vi "Kernel.vi"(0 "ref in":refnum<class "G#StaticClass.lvclass">, 1 "object name":string, 2 "option 1":bool, 3 "option 2":bool, 4 "depth":i32, 5 "error in (no error)":errorcluster, 6 "state":T3, 7 "option 3":bool, 8 "attributes in":variant[](array[variant]), 10 "class attributes in":variant[](array[variant])) -> (11 "class attributes out":variant[](array[variant]), 12 "class hierarchy":T1[](array[typedef]), 13 "attributes out":variant[](array[variant]), 14 "ref out":refnum<class "G#StaticClass.lvclass">, 15 "AttributeRefs":u32[](array[numeric]), 16 "static attribute ref":u32, 17 "output 1":bool, 18 "output 2":bool, 19 "error out":errorcluster)   [LabVIEW 2017, in "G#StaticClass.lvclass"]
doc: "Class kernel, creates and destroys the data value references of the class."
uses:
  G#StaticClass.lvclass
  <vilib>/addons/_AddQ/G#Object/utils/G#Object_State.ctl
  C:/Program Files/National Instruments/LabVIEW 2017/vi.lib/addons/_AddQ/G#Object/G#Object.lvclass
  <vilib>/addons/_AddQ/G#Object/utils/G#Object_ClassHierarchy.ctl
  protected/ClassAttributes.ctl
  ClassAttributesRef.ctl
  <vilib>/addons/_AddQ/G#Object/G#Object.lvclass
panel:
  in  "class attributes type":T2
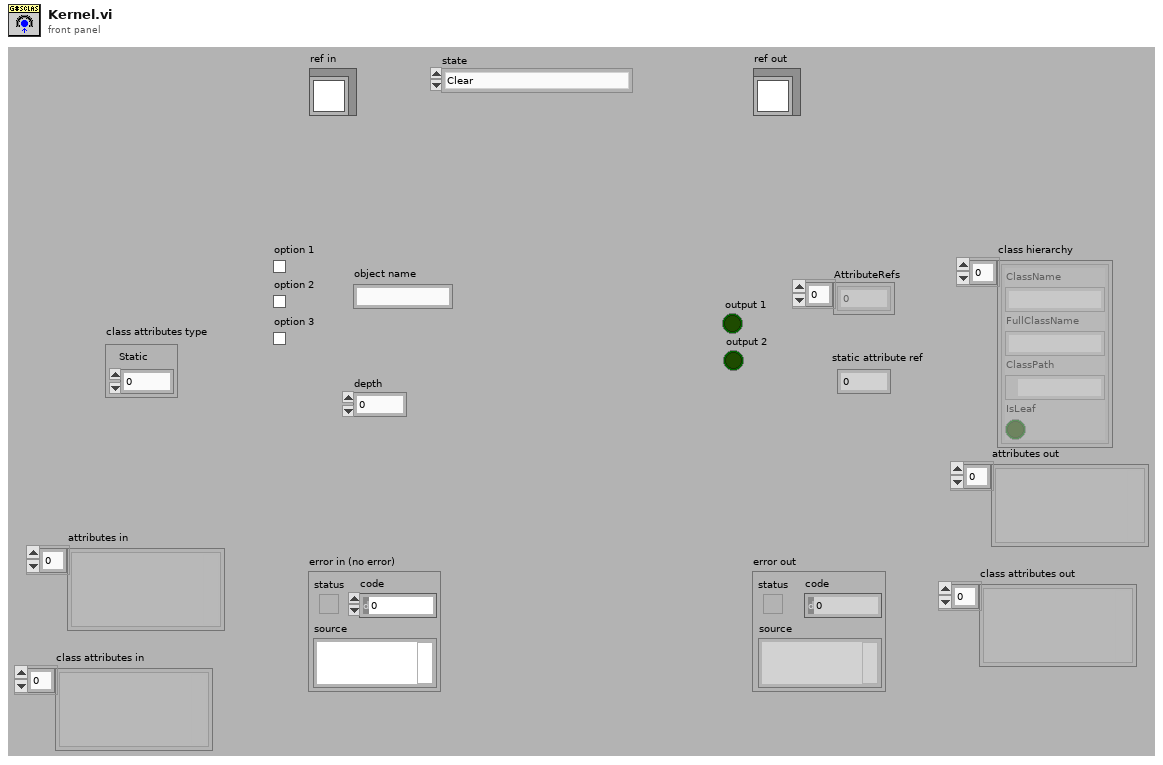
[diagram p1: front panel]
types:
  T1 = typedef "G#Object.lvclass/G#Object_ClassHierarchy.ctl" = cluster{"ClassName":string, "FullClassName":string, "ClassPath":path, "IsLeaf":bool}
  T2 = typedef "G#StaticClass.lvclass/ClassAttributes.ctl" = cluster{"Static":i32}
  T3 = typedef "G#Object.lvclass/G#Object_State.ctl" = enum16{"Clear", "Create", "Delete", "Get class attributes", "Class hierarchy", "Get attribute value", "Set attribute value"}
  T4 = typedef "G#StaticClass.lvclass/ClassAttributesRef.ctl" = refnum<data-value>
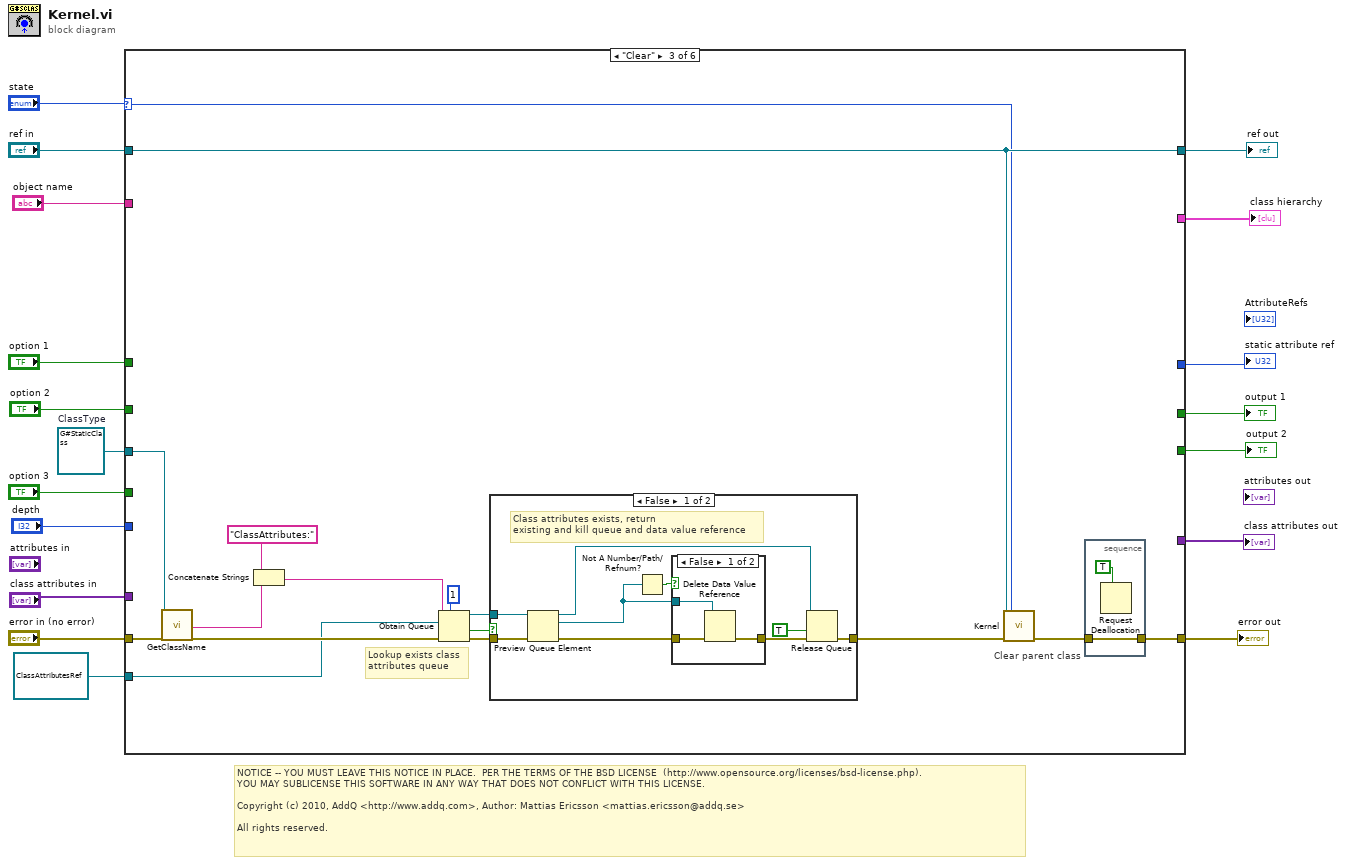
[diagram p0: block diagram]
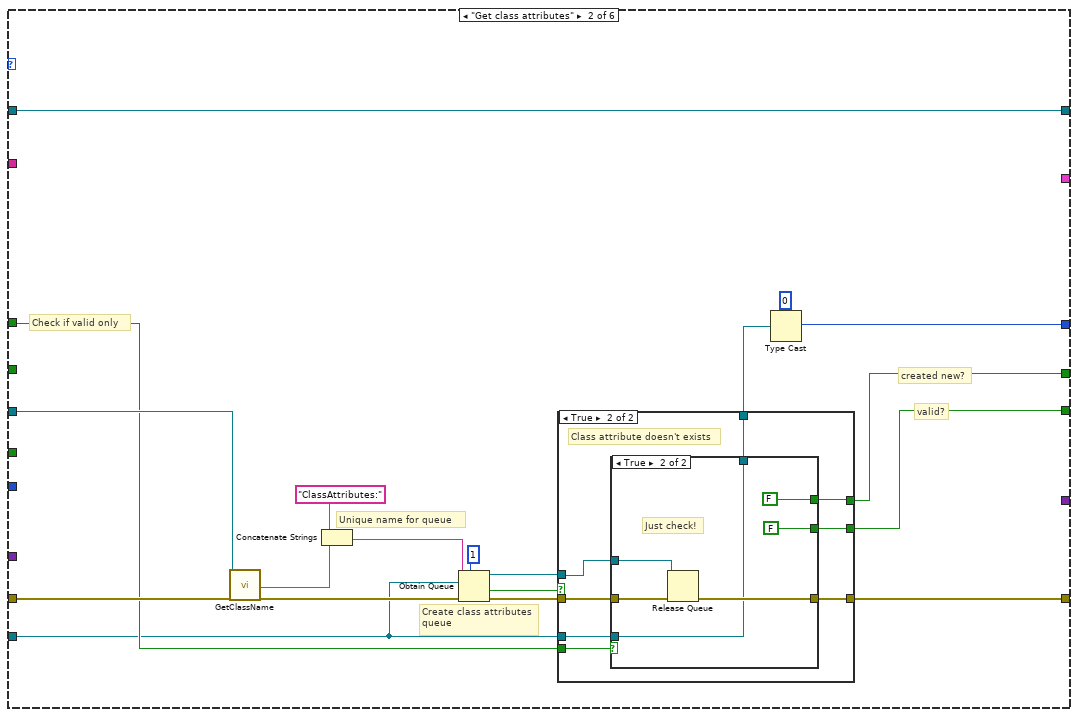
[diagram p3: hidden frame]
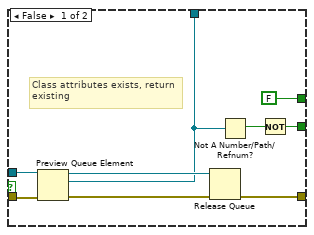
[diagram p4: hidden frame]
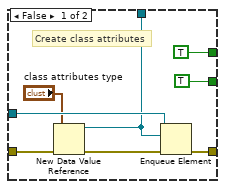
[diagram p5: hidden frame]
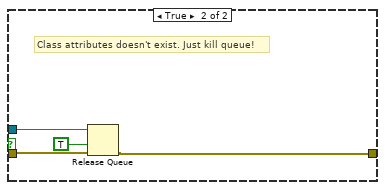
[diagram p7: hidden frame]
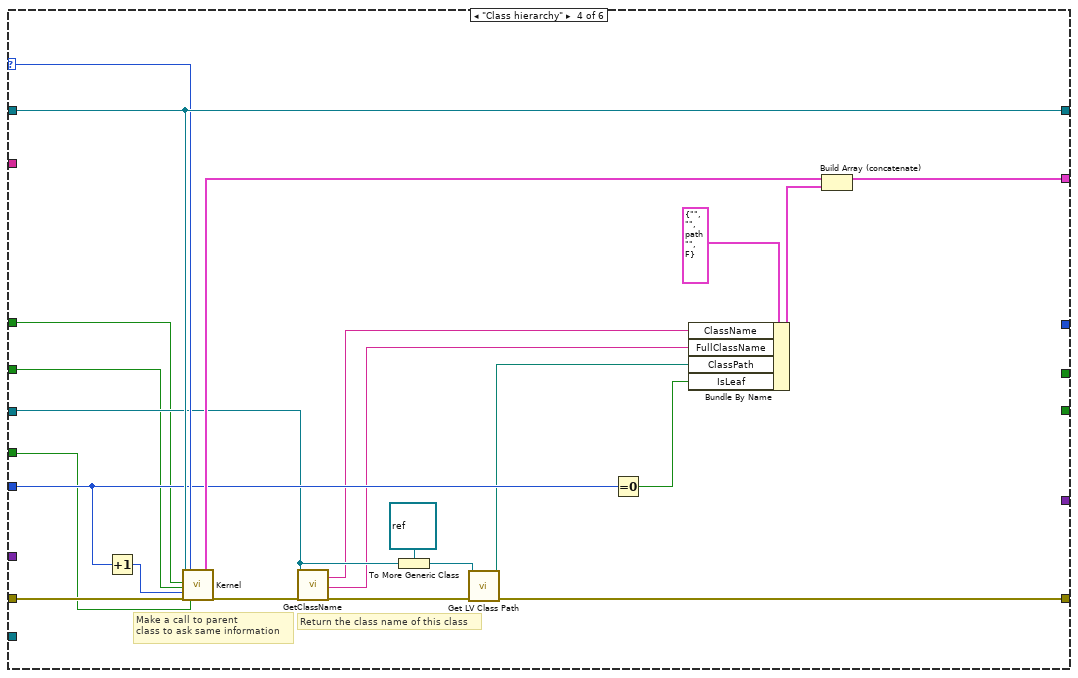
[diagram p8: hidden frame]
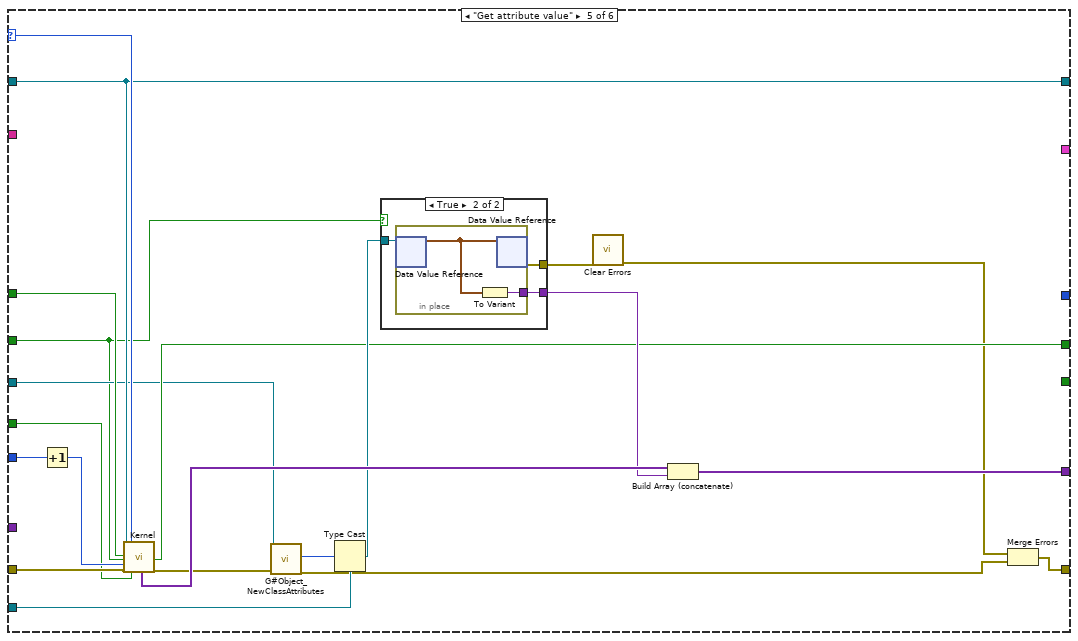
[diagram p9: hidden frame]
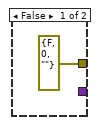
[diagram p10: hidden frame]
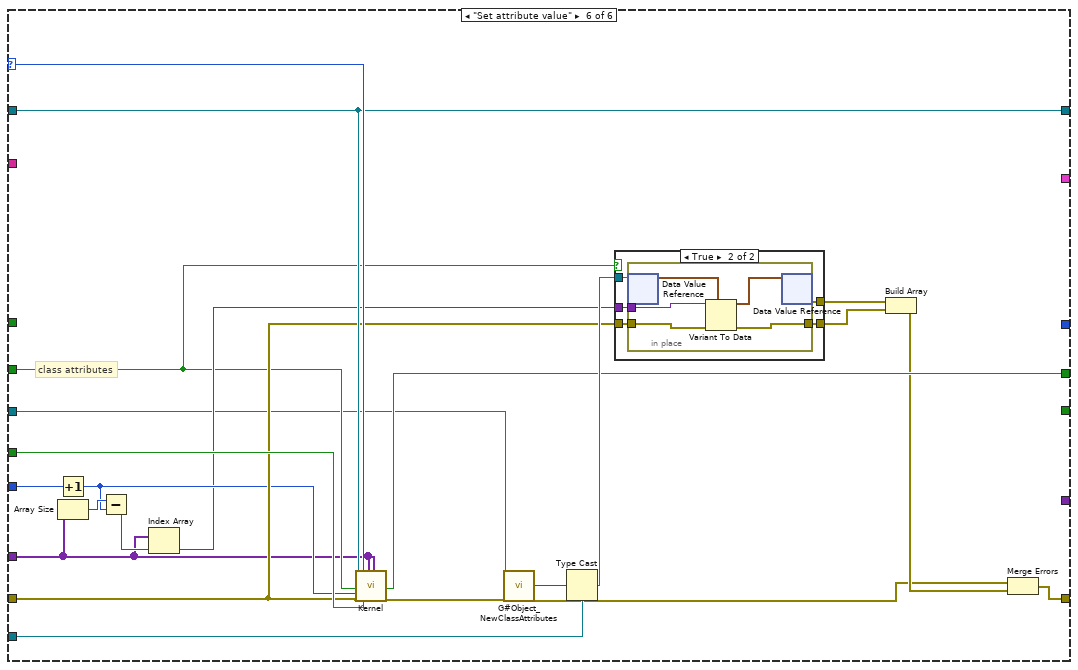
[diagram p11: hidden frame]
diagram:
  w8 = refnum<class "G#StaticClass.lvclass"> refnum  # ClassType
  # "NOTICE -- YOU MUST LEAVE THIS NOTICE IN PLACE.  PER THE TERMS OF THE BSD LICENSE  (http://www.opensource.org/licenses/bsd-license.php).\nYOU MAY SUBLICENSE THIS SOFTWARE IN ANY WAY THAT DOES NOT CONFLICT WITH THIS LICENSE.\n\nCopyright (c) 2010, AddQ <http://www.addq.com>, Author: Mattias Ericsson <mattias.ericsson@addq.se>\n\nAll rights reserved."
  n1 = case shown="\"Clear\"" "state" {
    selector: "state" -> [_ _ w74 w125 w148 w176]
    tunnel: "ref in" -> [w20 w39 w75 w126 w144 w175]
    tunnel: [w20 w39 w75 w126 w144 w175] -> w16
    tunnel: "error in (no error)" -> [w19 w38 w86 w111 w147 w169]
    tunnel: [w19 w28 w72 w109 w143 w174] -> w14
    tunnel: "depth" -> [_ _ _ w118 w138 w165]
    tunnel: "object name" -> [_ _ _ _ _ _]
    tunnel: "option 1" -> [_ w24 _ w108 w136 _]
    tunnel: [_ w21 _ _ w134 w170] -> w10
    tunnel: [_ w29 _ _ _ _] -> w9
    tunnel: w8 -> [_ w26 w77 w114 w132 w155]
    tunnel: T4 refnum ("data value reference") -> [_ w23 w76 _ w141 w173]
    tunnel: [_ _ _ w123 _ _] -> w6
    tunnel: [_ _ _ _ w145 _] -> w5
    tunnel: "option 2" -> [_ _ _ w107 w128 w160]
    tunnel: "option 3" -> [_ _ _ w106 w135 w171]
    tunnel: [_ w22 _ _ _ _] -> w2
    tunnel: "class attributes in" -> [_ _ _ _ _ w159]
    frame Default {
    }
    frame "Get class attributes" {
      # "valid?"
      # "created new?"
      # "Check if valid only"
      # "Unique name for queue"
      # "Create class attributes\nqueue"
      n2 = call-dynamic "GetClassName.vi"("reference in"=w26, "error in (no error)"=w38) -> ("full class name"=w27:string, "error out"=w33:errorcluster)  [unwired: 13 in, 3 out]
      n3 = Concatenate Strings("ClassAttributes:" ("string"), w27) -> (w32:string)
      n4 = Obtain Queue(max queue size (-1, unlimited)=1, name (unnamed)=w32, element data type=w23, error in (no error)=w33) -> (queue out=w34:refnum<queue>, created new?=w25:bool, error out=w35:errorcluster)  [unwired: 1 in]
      n5 = case shown="True" w25 {
        tunnel: w35 -> [w48 w56]
        tunnel: w34 -> [w47 w55]
        tunnel: [w46 w53] -> w28
        tunnel: [w42 w54] -> w30
        tunnel: w24 -> [_ w52]
        tunnel: w23 -> [_ w51]
        tunnel: [w41 w50] -> w22
        tunnel: [FALSE w49] -> w21
        frame False {
          # "Class attributes exists, return\nexisting"
          n6 = Preview Queue Element(queue=w47, error in (no error)=w48) -> (queue out=w44:refnum<queue>, element=w42:T4, error out=w45:errorcluster)  [unwired: 1 in, 1 out]
          n7 = Release Queue(queue=w44, error in (no error)=w45) -> (error out=w46:errorcluster)  [unwired: 1 in, 2 out]
          n8 = Not A Number/Path/Refnum?(number/path/refnum=w42) -> (NaN/Path/Refnum?=w40:bool)
          n9 = Not(x=w40) -> (.not. x?=w41:bool)
        }
        frame True {
          # "Class attribute doesn't exists"
          n10 = case shown="True" w52 {
            tunnel: w56 -> [w64 w70]
            tunnel: w55 -> [w62 w69]
            tunnel: [w61 w67] -> w54
            tunnel: [w60 w68] -> w53
            tunnel: w51 -> [_ w67]
            tunnel: [TRUE FALSE] -> w50
            tunnel: [TRUE FALSE] -> w49
            frame False {
              # "Create class attributes"
              n11 = New Data Value Reference(data value="class attributes type", error in=w64) -> (data value reference=w61:refnum<data-value>, error out=w63:errorcluster)
              n12 = Enqueue Element(queue=w62, element=w61, error in (no error)=w63) -> (error out=w60:errorcluster)  [unwired: 1 in, 2 out]
            }
            frame True {
              # "Just check!"
              n13 = Release Queue(queue=w69, error in (no error)=w70) -> (error out=w68:errorcluster)  [unwired: 1 in, 2 out]
            }
          }
        }
      }
      n14 = Type Cast(type=u32 0, x=w30) -> (*(type *) &x=w29:u32)
    }
    frame "Clear" {
      # "Clear parent class"
      # "Lookup exists class\nattributes queue"
      n15 = call-dynamic "GetClassName.vi"("reference in"=w77, "error in (no error)"=w86) -> ("full class name"=w78:string, "error out"=w80:errorcluster)  [unwired: 13 in, 3 out]
      n16 = Concatenate Strings("ClassAttributes:" ("string"), w78) -> (w79:string)
      n17 = Obtain Queue(max queue size (-1, unlimited)=1, name (unnamed)=w79, element data type=w76, error in (no error)=w80) -> (queue out=w81:refnum<queue>, created new?=w82:bool, error out=w83:errorcluster)  [unwired: 1 in]
      n18 = case shown="False" w82 {
        tunnel: w83 -> [w92 w104]
        tunnel: w81 -> [w93 w105]
        tunnel: [w95 w103] -> w73
        frame False {
          # "Class attributes exists, return\nexisting and kill queue and data value reference"
          n19 = Preview Queue Element(queue=w93, error in (no error)=w92) -> (queue out=w90:refnum<queue>, element=w89:T4, error out=w91:errorcluster)  [unwired: 1 in, 1 out]
          n20 = Not A Number/Path/Refnum?(number/path/refnum=w89) -> (NaN/Path/Refnum?=w96:bool)
          n21 = case shown="False" w96 {
            tunnel: w91 -> [w100 w101]
            tunnel: [w99 w101] -> w94
            tunnel: w89 -> [w98 _]
            frame False {
              n22 = Delete Data Value Reference(data value reference=w98, error in=w100) -> (error out=w99:errorcluster)  [unwired: 1 out]
            }
            frame True {
            }
          }
          n23 = Release Queue(queue=w90, force destroy? (F)=TRUE, error in (no error)=w94) -> (error out=w95:errorcluster)  [unwired: 2 out]
        }
        frame True {
          # "Class attributes doesn't exist. Just kill queue!"
          n24 = Release Queue(queue=w105, force destroy? (F)=TRUE, error in (no error)=w104) -> (error out=w103:errorcluster)  [unwired: 2 out]
        }
      }
      n25 = call-parent "Kernel.vi"("reference in"=w75, "error in (no error)"=w73, "state"=w74) -> ("error out"=w71:errorcluster)  [unwired: 8 in, 8 out]
      n26 = stacked-sequence {
        tunnel: w71 -> [w87]
        tunnel: [w87] -> w72
        frame #0 {
          n27 = Request Deallocation(TRUE ("flag")) -> ()
        }
      }
    }
    frame "Class hierarchy" {
      # "Make a call to parent\nclass to ask same information"
      # "Return the class name of this class"
      n28 = Increment(x=w118) -> (x+1=w119:i32)
      n29 = call-parent "Kernel.vi"("reference in"=w126, "option 1"=w108, "option 2"=w107, "depth"=w119, "error in (no error)"=w111, "state"=w125, "option 3"=w106) -> ("class hierarchy"=w124:T1[], "error out"=w110:errorcluster)  [unwired: 4 in, 7 out]
      n30 = call-dynamic "GetClassName.vi"("reference in"=w114, "error in (no error)"=w110) -> ("class name"=w112:string, "full class name"=w113:string, "error out"=w115:errorcluster)  [unwired: 13 in, 2 out]
      n31 = To More Generic Class(target class=refnum<class> refnum ("object"), reference=w114) -> (generic class reference=w120:refnum<class>)
      n32 = call <vilib>:"Get LV Class Path.vi"("error in (no error)"=w115, "object"=w120) -> ("error out"=w109:errorcluster, "class path"=w116:path)  [unwired: 8 in]
      n33 = Equal To 0?(x=w118) -> (x = 0?=w117:bool)
      n34 = Bundle By Name(cluster=T1 {"ClassName"="", "FullClassName"="", "ClassPath"=path "", "IsLeaf"=FALSE} ("ClassHierarchy"), "ClassName"=w112, "FullClassName"=w113, "ClassPath"=w116, "IsLeaf"=w117) -> (w121:T1)
      n35 = Build Array (concatenate)(w124, w121) -> (w123:T1[])
    }
    frame "Get attribute value" {
      n36 = Increment(x=w138) -> (x+1=w137:i32)
      n37 = call-parent "Kernel.vi"("reference in"=w144, "option 1"=w136, "option 2"=w128, "depth"=w137, "error in (no error)"=w147, "state"=w148, "option 3"=w135) -> ("class attributes out"=w146:variant[], "output 1"=w134:bool, "error out"=w133:errorcluster)  [unwired: 4 in, 6 out]
      n38 = call <vilib>:"G#Object_NewClassAttributes.vi"("reference in"=w132, "error in (no error)"=w133) -> ("static attribute ref"=w131:u32, "error out"=w129:errorcluster)  [unwired: 13 in, 3 out]
      n39 = Type Cast(type=w141, x=w131) -> (*(type *) &x=w140:T4)
      n40 = case shown="True" w128 {
        tunnel: [errorcluster {"status"=FALSE, "code"=0, "source"=""} ("error IO") w152] -> w142
        tunnel: w140 -> [_ w151]
        tunnel: [_ w150] -> w139
        frame False {
        }
        frame True {
          n41 = in-place {
            in-place-border: [w154] -> w150
            n42 = in-place-dvr #1(w151) -> (w153:T2)  [unwired: 1 out]
            n43 = To Variant(anything=w153) -> (Variant=w154:variant)
            n44 = in-place-dvr #1(w153) -> (w152:errorcluster)  [unwired: 1 out]
          }
        }
      }
      n45 = call <vilib>:"Clear Errors.vi"("error in (no error)"=w142) -> ("error out"=w130:errorcluster)  [unwired: 5 in, 1 out]
      n46 = Build Array (concatenate)(w146, w139) -> (w145:variant[])
      n47 = Merge Errors(w130, w129) -> (w143:errorcluster)
    }
    frame "Set attribute value" {
      # "class attributes"
      n48 = Increment(x=w165) -> (x+1=w163:i32)
      n49 = Array Size(array=w159) -> (size(s)=w164:i32)
      n50 = Subtract(x=w164, y=w163) -> (x-y=w162:i32)
      n51 = Index Array(array=w159, index=w162) -> (element=w161:variant)
      n52 = call-parent "Kernel.vi"("reference in"=w175, "option 2"=w160, "depth"=w163, "error in (no error)"=w169, "state"=w176, "option 3"=w171, "attributes in"=w159, "class attributes in"=w159) -> ("output 1"=w170:bool, "error out"=w158:errorcluster)  [unwired: 3 in, 7 out]
      n53 = call <vilib>:"G#Object_NewClassAttributes.vi"("reference in"=w155, "error in (no error)"=w158) -> ("static attribute ref"=w156:u32, "error out"=w157:errorcluster)  [unwired: 13 in, 3 out]
      n54 = Type Cast(type=w173, x=w156) -> (*(type *) &x=w172:T4)
      n55 = case shown="True" w160 {
        tunnel: w172 -> [_ w182]
        tunnel: w169 -> [w177 w181]
        tunnel: [w177 w180] -> w168
        tunnel: [w177 w179] -> w167
        tunnel: w161 -> [_ w178]
        frame False {
        }
        frame True {
          n56 = in-place {
            in-place-border: w181 -> [w185]
            in-place-border: [w184] -> w179
            in-place-border: w178 -> [w183]
            n57 = in-place-dvr #2(w182) -> (w187:T2)  [unwired: 1 out]
            n58 = Variant To Data(error in=w185, type=w187, Variant=w183) -> (data=w186:T2, error out=w184:errorcluster)
            n59 = in-place-dvr #2(w186) -> (w180:errorcluster)  [unwired: 1 out]
          }
        }
      }
      n60 = Build Array(w168, w167) -> (w166:errorcluster[])
      n61 = Merge Errors(w157, w166) -> (w174:errorcluster)
    }
  }
  "error out" <- w14
  "ref out" <- w16
  "static attribute ref" <- w9
  "output 1" <- w10
  "output 2" <- w2
  "class hierarchy" <- w6
  "class attributes out" <- w5
